vi "OpenDefaultConfigFile.vi"(8 "error in (no error)":errorcluster, 11 "Device in":refnum<class "Device.lvclass">) -> (0 "error out":errorcluster, 2 "refnum":T1, 3 "Device out":refnum<class "Device.lvclass">)   [LabVIEW 2020, in "Device.lvlib" / "Device.lvclass"]
uses:
  Device.lvclass
  <vilib>/Utility/config.llb/Config Data RefNum.ctl
  Device.lvclass/Device.ctl
  <vilib>/Utility/config.llb/NI_LVConfig.lvlib
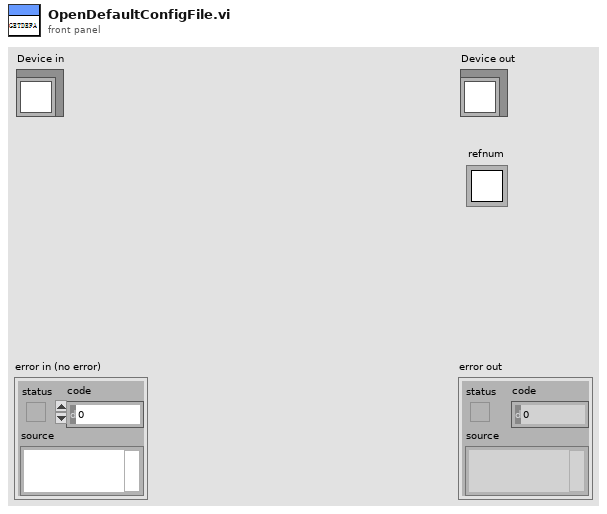
[diagram p1: front panel]
types:
  T1 = typedef "NI_LVConfig.lvlib/Config Data RefNum.ctl" = refnum<k1>
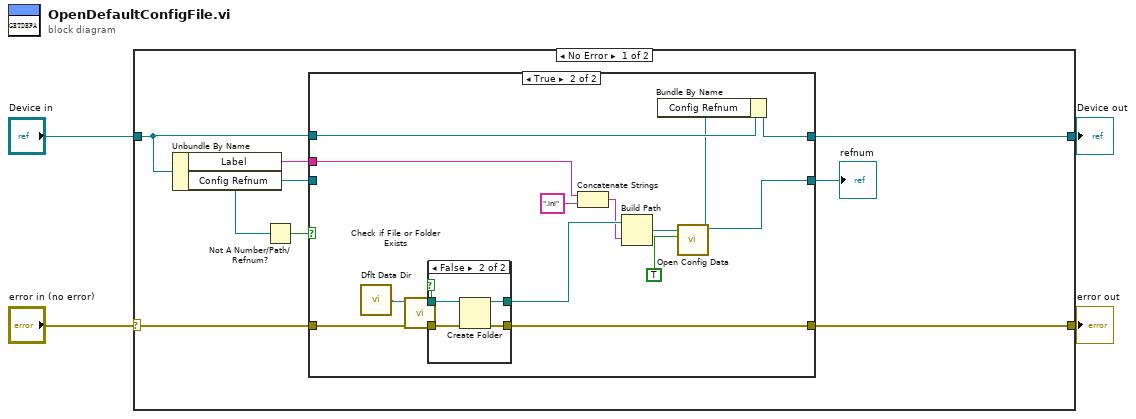
[diagram p0: block diagram]
diagram:
  n1 = case shown="No Error" "error in (no error)" {
    selector: "error in (no error)" -> [w12 w38]
    tunnel: [w11 w38] -> w3
    tunnel: [w8 w37] -> w1
    tunnel: "Device in" -> [w10 w37]
    frame No Error {
      n2 = Unbundle By Name(w10) -> ("Label"=w9:string, "Config Refnum"=w5:T1)
      n3 = Not A Number/Path/Refnum?(number/path/refnum=w5) -> (NaN/Path/Refnum?=w7:bool)
      n4 = case shown="True" w7 {
        tunnel: w12 -> [w14 w25]
        tunnel: [w14 w24] -> w11
        tunnel: w10 -> [w15 w23]
        tunnel: w9 -> [_ w22]
        tunnel: [w15 w17] -> w8
        tunnel: [w13 w16] -> w6
        tunnel: w5 -> [w13 _]
        frame False {
        }
        frame True {
          n5 = call <vilib>:"Dflt Data Dir.vi"() -> ("App:Default Data Directory"=w27:path)
          n6 = call <vilib>:"Check if File or Folder Exists.vi"("error in (no error)"=w25, "path"=w27) -> ("error out"=w29:errorcluster, "file or folder exists?"=w28:bool, "dup path"=w30:path)  [unwired: 7 in]
          n7 = case shown="False" w28 {
            tunnel: w29 -> [w31 w36]
            tunnel: w30 -> [w32 w35]
            tunnel: [w31 w34] -> w24
            tunnel: [w32 w33] -> w26
            frame True {
            }
            frame False {
              n8 = Create Folder(path (use dialog)=w35, error in=w36) -> (created path=w33:path, error out=w34:errorcluster)  [unwired: 1 in, 1 out]
            }
          }
          n9 = Concatenate Strings(w22, ".ini" ("string")) -> (w20:string)
          n10 = Build Path(base path=w26, name or relative path=w20) -> (appended path=w18:path)
          n11 = call <vilib>:"Open Config Data.vi"("create file if necessary (T)"=TRUE, "configuration file path"=w18) -> ("refnum"=w16:T1)  [unwired: 7 in, 2 out]
          n12 = Bundle By Name(cluster=w23, "Config Refnum"=w16) -> (w17:refnum<class "Device.lvclass">)
        }
      }
      "refnum" <- w6
    }
    frame Error {
    }
  }
  "error out" <- w3
  "Device out" <- w1
